vi "Menu List - Top Level VI.vi"(6 "stop":bool, 7 "Add to list":bool, 10 "Combo Box":string(combo)) -> ()   [LabVIEW 2012]
doc: "This VI demonstrates how to progrommatically edit the list of items within a combo Box"
panel:
  # "Overview: This example VI demonstrates how o programmatically edit the list of items within a combo Box.\nRequirements: LabVIEW 2012 or compatible\nInstructions:\n1. Run this VI\n2. Click on Edit List and modify the elements in the Combo Box \n3. Stop the VI"
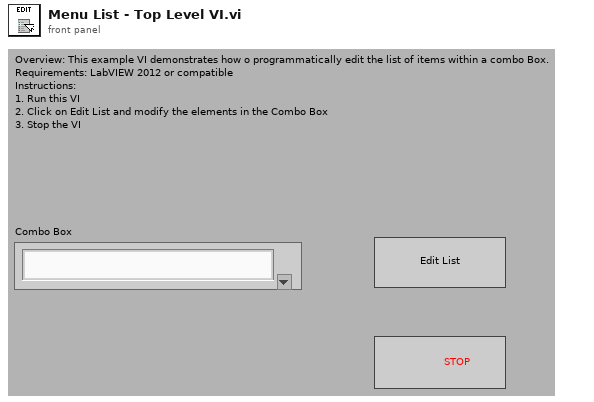
[diagram p1: front panel]
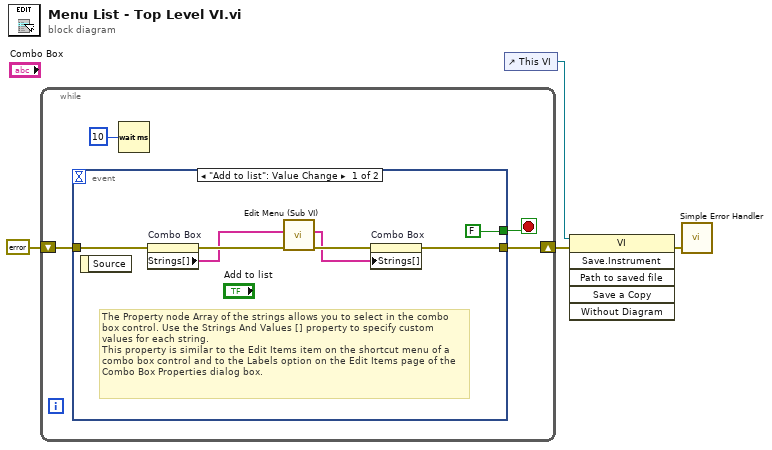
[diagram p0: block diagram]
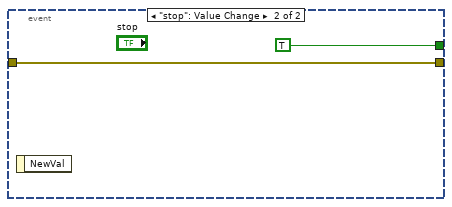
[diagram p2: hidden frame]
diagram:
  n1 = while {
    shift-right: [w6] -> w3
    shift-left: errorcluster {"status"=FALSE, "code"=0, "source"=""} ("error out") -> [w5]
    stop <- w7 stop-if-true
    n2 = event shown="[0] \"Add to list\": Value Change" {
      selector: _ -> [_ _]
      dyn-events: _ -> [_ _]
      timeout: _ -> [_ _]
      tunnel: [FALSE TRUE] -> w7
      tunnel: [w14 w16] -> w6
      tunnel: w5 -> [w13 w16]
      event "Add to list": Value Change {
        # "The Property node Array of the strings allows you to select in the combo box control. Use the Strings And Values [] property to specify custom values for each string.\nThis property is similar to the Edit Items item on the shortcut menu of a combo box control and to the Labels option on the Edit Items page of the Combo Box Properties dialog box."
        n3 = event-data() -> ()  [unwired: 2 out]
        n4 = property on="Combo Box" class="CmbBox"(error in=w13) -> (error out=w12:errorcluster, "Strings[]"=w11:string[])  [unwired: 1 in, 1 out]
        n5 = call "Edit Menu (Sub VI).vi"("error in (no error)"=w12, "Add/remove"=w11) -> ("error out"=w10:errorcluster, "Add/remove 2"=w9:string[])  [unwired: 8 in]
        n6 = property on="Combo Box" class="CmbBox"(error in=w10, "Strings[]"=w9) -> (error out=w14:errorcluster)  [unwired: 1 in, 1 out]
      }
      event "stop": Value Change {
        n7 = event-data() -> ()  [unwired: 2 out]
      }
    }
    n8 = Wait (ms)(milliseconds to wait=u32 10) -> ()  [unwired: 1 out]
  }
  n9 = control-ref of="This VI"() -> (w4:refnum<vi>)
  n10 = invoke class="VI" method="Save.Instrument"(reference=w4, error in=w3) -> (error out=w1:errorcluster)  [unwired: 4 in, 5 out]
  n11 = call <vilib>:"Simple Error Handler.vi"("error in (no error)"=w1) -> ()  [unwired: 4 in, 5 out]
